vi "直方图均衡化.vi"() -> ()   [LabVIEW 2018]
uses:
  <vilib>/vision/NI_Vision_Development_Module.lvlib
panel:
  out "波形图 3":T1(graph)
  out "Image 3":T2(plugin-control)
  out "波形图 2":T1(graph)
  out "Image 2":T2(plugin-control)
  out "error out":errorcluster
  out "波形图":T1(graph)
  out "Image":T2(plugin-control)
  in  "路径":path
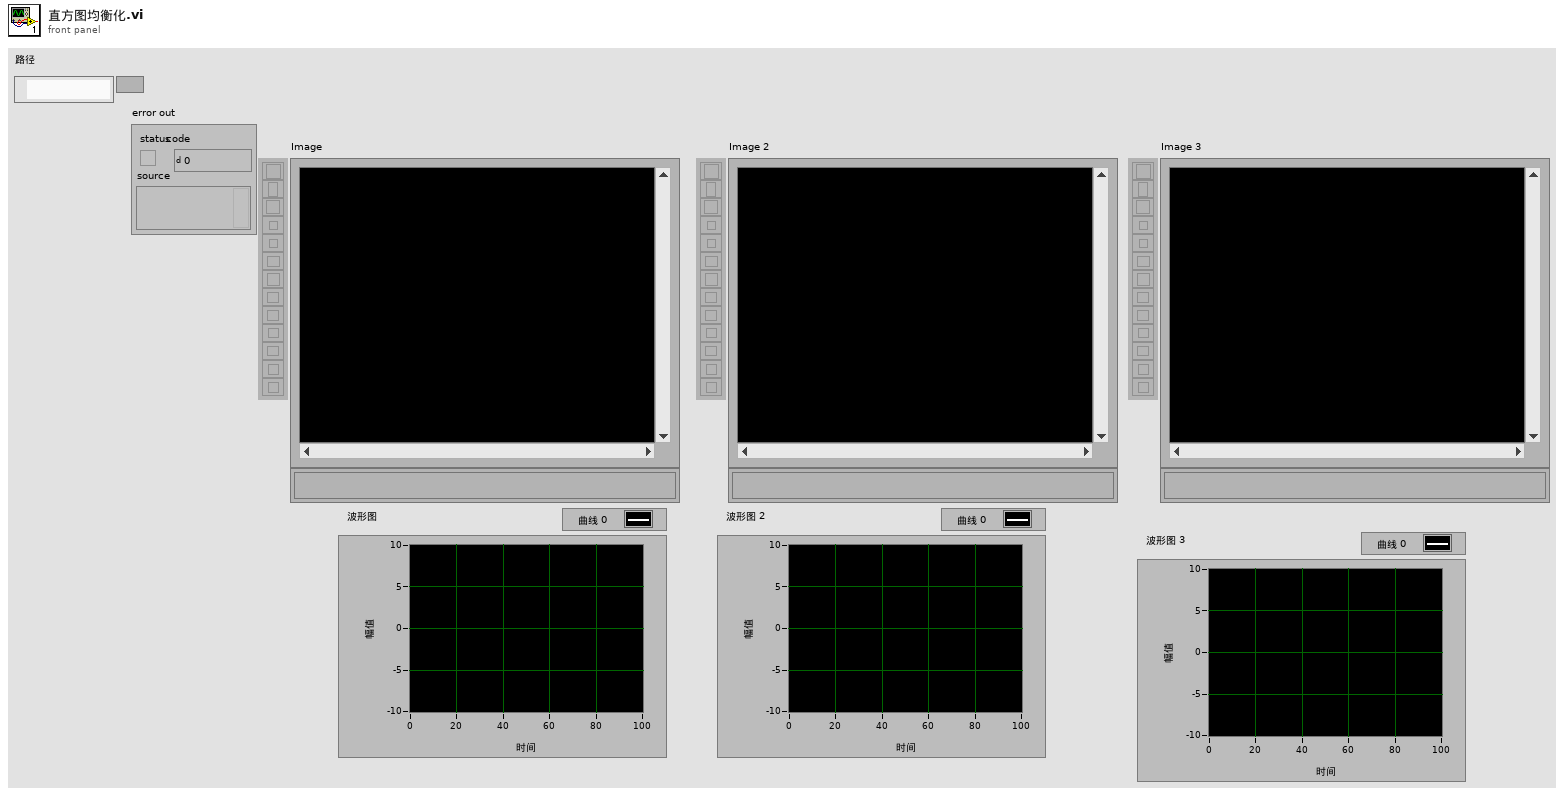
[diagram p1: front panel]
types:
  T1 = cluster{"Starting Value":sgl, "Incremental Value":sgl, "Histogram":u32[]}
  T2 = typedef "IMAQ Image.ctl" = refnum<image>
  T3 = cluster{"histogram":u32[], "Minimal Value":sgl, "Maximal Value":sgl, "Starting Value":sgl, "Interval Width":sgl, "Mean Value":sgl, "Standard  Variation":sgl, "Area (pixels)":i32}
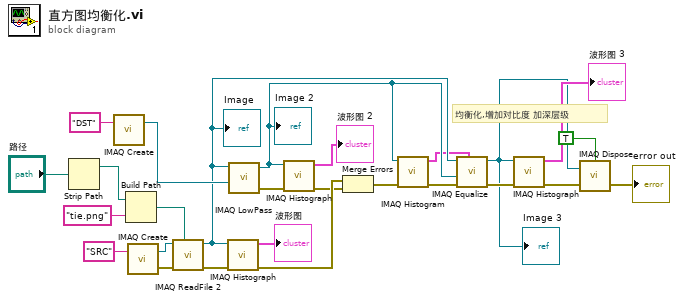
[diagram p0: block diagram]
diagram:
  # "均衡化,增加对比度 加深层级"
  n1 = Strip Path(path="路径") -> (stripped path=w25:path)  [unwired: 1 out]
  n2 = call "IMAQ Create"("Image Name"="DST") -> ("New Image"=w15:T2)  [unwired: 4 in, 1 out]
  n3 = Build Path(base path=w25, name or relative path="tie.png" ("名称或相对路径")) -> (appended path=w21:path)
  n4 = call "IMAQ Create"("Image Name"="SRC") -> ("New Image"=w23:T2, "error out"=w22:errorcluster)  [unwired: 4 in]
  n5 = call "IMAQ ReadFile 2"("File Path"=w21, "error in (no error)"=w22, "Image"=w23) -> ("error out"=w19:errorcluster, "Image Out"=w12:T2)  [unwired: 4 in, 3 out]
  "Image" <- w12
  n6 = call "IMAQ Histograph"("error in (no error)"=w19, "Image"=w12) -> ("error out"=w10:errorcluster, "Histogram Graph"=→"波形图":T1)  [unwired: 6 in, 2 out]
  n7 = call "IMAQ LowPass"("Image Src"=w12, "Image Dst"=w15) -> ("Image Dst Out"=w11:T2, "error out"=w14:errorcluster)  [unwired: 5 in]
  "Image 2" <- w11
  n8 = call "IMAQ Histograph"("error in (no error)"=w14, "Image"=w11) -> ("error out"=w9:errorcluster, "Histogram Graph"=→"波形图 2":T1)  [unwired: 6 in, 2 out]
  n9 = Merge Errors(w10, w9) -> (w8:errorcluster)
  n10 = call "IMAQ Histogram"("error in (no error)"=w8, "Image"=w11) -> ("error out"=w7:errorcluster, "Histogram Report"=w6:T3)  [unwired: 8 in]
  n11 = call "IMAQ Equalize"("Histogram Report"=w6, "error in (no error)"=w7, "Image Dst"=w11, "Image Src"=w12) -> ("error out"=w5:errorcluster, "Image Dst Out"=w3:T2)  [unwired: 6 in]
  "Image 3" <- w3
  n12 = call "IMAQ Histograph"("error in (no error)"=w5, "Image"=w3) -> ("error out"=w2:errorcluster, "Histogram Graph"=→"波形图 3":T1)  [unwired: 6 in, 2 out]
  n13 = call "IMAQ Dispose"("All Images? (No)"=TRUE, "Image"=w3, "error in (no error)"=w2) -> ("error out"=→"error out":errorcluster)  [unwired: 3 in]
